vi "Close.vi"(8 "error in (no error)":errorcluster, 11 "Abstract Power Supply in":refnum<class "Abstract Power Supply.lvclass">) -> (0 "error out":errorcluster, 3 "Abstract Power Supply out":refnum<class "Abstract Power Supply.lvclass">)   [LabVIEW 2014, in "Generic Power Supply.lvlib" / "Abstract Power Supply.lvclass"]
uses:
  Abstract Power Supply.lvclass
  Generic Instrument/Generic Instrument.lvclass
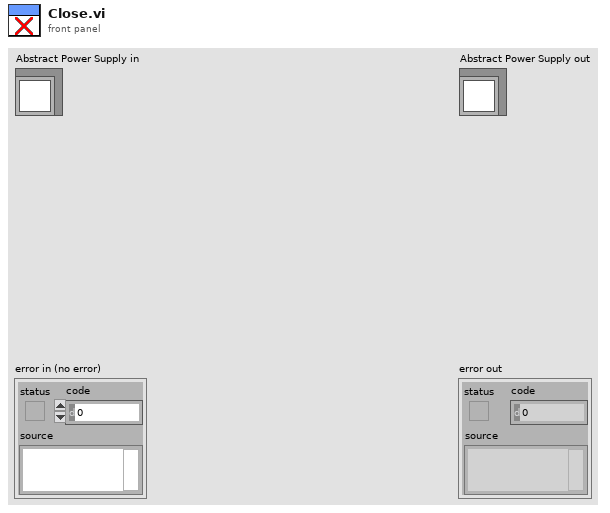
[diagram p1: front panel]
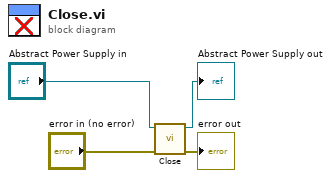
[diagram p0: block diagram]
diagram:
  n1 = call-parent "Close.vi"("error in (no error)"="error in (no error)", "Generic Instrument in"="Abstract Power Supply in") -> ("error out"=→"error out":errorcluster, "Generic Instrument out"=→"Abstract Power Supply out":refnum<class "Abstract Power Supply.lvclass">)  [unwired: 8 in]
